vi "Write Multiple Registers Response.vi"(8 "error in (no error)":errorcluster, 9 "Modbus Data Unit in":T1={"function"=1, "Data"=[]} {"function" items=["Read Discrete Inputs"=2, "Read Coils"=1, "Write Single Coil"=5, "Write Multiple Coils"=15, "Read Input Register"=4, "Read Holding Registers"=3, "Write Single Register"=6, "Write Multiple Registers"=16, "Read/Write Multiple Registers"=23, "Mask Write Register"=22, "Read FIFO Queue"=24, "Read File Record"=20, "Write File Record"=21, "Read Exception Status"=7, "Diagnostic"=8, "Get Com Event Counter"=11, "Get Com Event Log"=12, "Report Slave ID"=17, "Read Device Identification"=43]; "Data" format="%.0x"}) -> (0 "error out":errorcluster, 1 "number of registers":u16, 2 "start address":u16)   [LabVIEW 2021, in "NI_modbus_upd.lvlib"]
uses:
  NI_modbus_upd.lvlib
  Ctl/MB Modbus Data Unit.ctl
  Modbus Data Unit (PDU)/Function.ctl
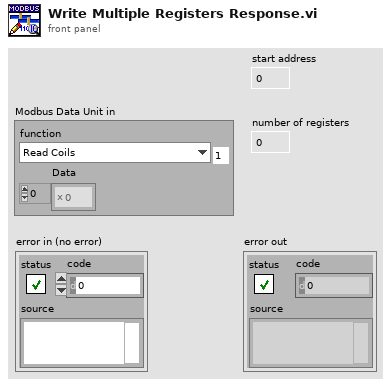
[diagram p1: front panel]
types:
  T1 = typedef "NI_modbus_upd.lvlib/MB Modbus Data Unit.ctl" = cluster{"function":T2, "Data":u8[]}
  T2 = typedef "NI_modbus_upd.lvlib/Function.ctl" = u8
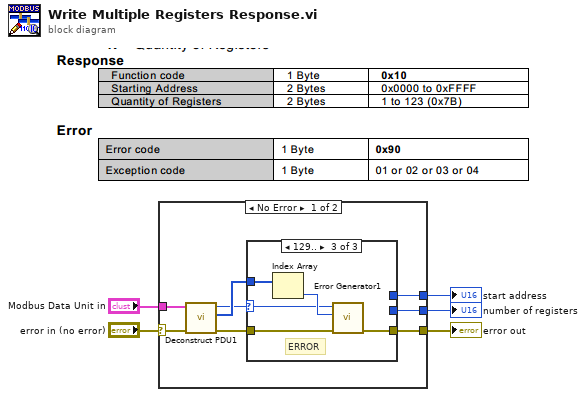
[diagram p0: block diagram]
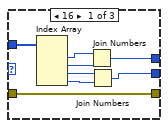
[diagram p2: hidden frame]
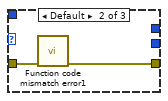
[diagram p3: hidden frame]
diagram:
  n1 = case shown="No Error" "error in (no error)" {
    selector: "error in (no error)" -> [w12 w29]
    tunnel: [w13 w29] -> w4
    tunnel: "Modbus Data Unit in" -> [w6 _]
    tunnel: [w9 _] -> w3
    tunnel: [w8 _] -> w2
    frame No Error {
      n2 = call "Deconstruct PDU1.vi"("error in (no error)"=w12, "Modbus Data Unit in"=w6) -> ("error out"=w10:errorcluster, "data"=w11:u8[], "function"=w7:T2)  [unwired: 7 in]
      n3 = case shown="129.." w7 {
        selector: w7 -> [_ _ w24]
        tunnel: w10 -> [w20 w22 w25]
        tunnel: w11 -> [w21 _ w28]
        tunnel: [w20 w23 w27] -> w13
        tunnel: [w19 _ _] -> w9
        tunnel: [w18 _ _] -> w8
        frame 16 {
          n4 = Index Array(array=w21) -> (element #1=w17:u8, element #2=w16:u8, element #3=w15:u8, element #4=w14:u8)  [unwired: 4 in]
          n5 = Join Numbers(hi=w17, lo=w16) -> ((hi.lo)=w19:u16)
          n6 = Join Numbers(hi=w15, lo=w14) -> ((hi.lo)=w18:u16)
        }
        frame Default {
          n7 = call "Function code mismatch error1.vi"("error in (no error)"=w22) -> ("error out"=w23:errorcluster)  [unwired: 10 in]
        }
        frame 129.. {
          # "ERROR"
          n8 = Index Array(array=w28) -> (element=w26:u8)  [unwired: 1 in]
          n9 = call "Error Generator1.vi"("error in (no error)"=w25, "data return (error code)"=w26, "function return"=w24) -> ("error out"=w27:errorcluster)  [unwired: 8 in]
        }
      }
    }
    frame Error {
    }
  }
  "error out" <- w4
  "number of registers" <- w2
  "start address" <- w3
